vi "Download Confrigurations.vi"() -> ()   [LabVIEW 2024]
panel:
  in  "Tab Control":enum32{"BASIC CONFIGS", "Page 2"}(tab)
  out "DMM":string
  out "Power_Supply":string
  out "Application_Log":string
  out "Error_Log":string
  out "DB Config":string
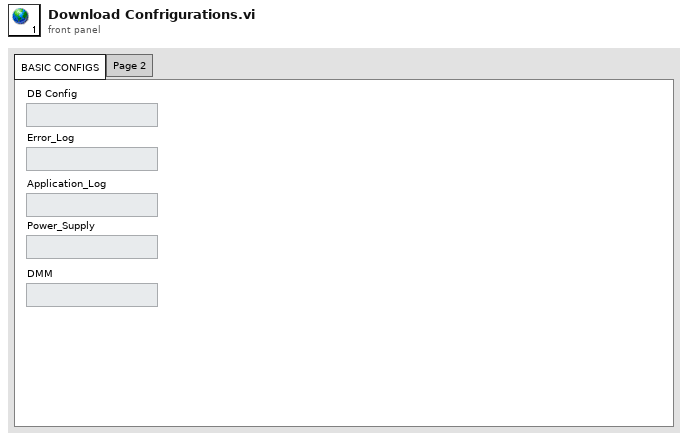
[diagram p1: front panel]
diagram:
